vi "ConfigUI.vi"() -> ()   [LabVIEW 2017, in "ThreePhasePLL editor node.lvclass"]
uses:
  ThreePhasePLL editor node.lvclass
  <vilib>/NI/Configuration Framework/Node/NodeRef.ctl
  <vilib>/NI/Configuration Framework/Node/NISE_CEF_Node.lvclass
  <vilib>/NI/AMC/Message Queue.ctl
  <vilib>/NI/AMC/Message.ctl
  <vilib>/NI/Tools/Keyed Array/KeyedArray.ctl
  <vilib>/NI/Configuration Framework/Node/UserEventRef.ctl
  <vilib>/NI/Configuration Framework/Controls/EventCluster.ctl
  <vilib>/NI/Configuration Framework/Node/RefreshUIEvent.ctl
  <vilib>/NI/Configuration Framework/Node/CacheState.ctl
  <vilib>/NI/Configuration Framework/Node/StopEvent.ctl
  <vilib>/NI/Configuration Framework/Node/NodeChangeEvent.ctl
  <vilib>/NI/DCAF/Tag Editor Core/control module/configuration/error classification setting.ctl
  <vilib>/NI/Tag Bus Module Framework/runtime/error classification.ctl
  <vilib>/NI/DCAF/Tag Editor Core/Table API/Available Tag Menu/channel action event.ctl
  <vilib>/NI/DCAF/Tag Editor Core/Table API/Available Tag Menu/dialog output action.ctl
  <vilib>/NI/Tag Bus Module Framework/channel/TBM channel.lvclass
  <vilib>/NI/Tag Bus/tag/tag descriptor.lvclass
  <vilib>/NI/DCAF/Tag Editor Core/Table API/Table Manager/Call Back Ref Type Def.ctl
  <vilib>/NI/DCAF/Tag Editor Core/Configuration Editor/Classes/Engine Parent/Engine Parent Editor Node.lvclass
  <vilib>/NI/DCAF/Tag Editor Core/Configuration Editor/Classes/Module editor node/module editor node.lvclass
  C:/Program Files (x86)/National Instruments/LabVIEW 2017/vi.lib/NI/Configuration Framework/serializable node/NISE_CEF_serializable node.lvclass
  <vilib>/rvi/Analysis/control/PID/Typedef/niFpgaPID_PIGains.ctl
  <vilib>/rvi/Analysis/control/PID/Typedef/niFpgaPID_OutputRange.ctl
  <vilib>/NI/DCAF/Tag Editor Core/Table API/Table Manager/references.ctl
  <vilib>/NI/DCAF/Tag Editor Core/Table API/Table Manager/Menu Definition.ctl
  <vilib>/NI/DCAF/Tag Editor Core/Table API/Table Manager/Menu Options.ctl
  <vilib>/NI/DCAF/Tag Editor Core/control module/configuration/control module configuration.lvclass
  C:/Program Files (x86)/National Instruments/LabVIEW 2017/vi.lib/NI/Configuration Framework/serializable configuration/NISE_CEF_serializable configuration.lvclass
  <vilib>/NI/DCAF/Tag Editor Core/control module/editor node/control module editor.lvclass
  module/configuration/ThreePhasePLL configuration.lvclass
  C:/Program Files (x86)/National Instruments/LabVIEW 2017/vi.lib/NI/DCAF/Tag Editor Core/control module/configuration/control module configuration.lvclass
  module/configuration/ThreePhasePLL configuration.lvclass/ThreePhasePLL configuration.ctl
  <vilib>/NI/DCAF/Tag Editor Core/control module/configuration/control module configuration.lvclass/control module configuration.ctl
  <vilib>/NI/Configuration Framework/serializable configuration/NISE_CEF_serializable configuration.lvclass/NISE_CEF_serializable configuration.ctl
  <vilib>/NI/PowerElectronicsControl/ThreePhasePLL/Interface/Configuration.ctl
  <vilib>/NI/Tag Bus Module Framework/channel/channel classification.ctl
  <vilib>/NI/DCAF/Tag Editor Core/control module/configuration/Write error classifications.vi
  <vilib>/NI/Tag Bus Module Framework/module configuration/TBM module configuration.lvclass
  <vilib>/NI/DCAF/Tag Editor Core/Configuration Editor/Classes/Module editor node/Read Module Configuration.vi
  <vilib>/NI/DCAF/Tag Editor Core/control module/editor node/read fixed channel configuration.vi
  <vilib>/Utility/LVClass/Get LV Class Name.vi
  <vilib>/NI/Configuration Framework/error generator/NISE_error generator.vi
  <vilib>/NI/Configuration Framework/serializable configuration/NISE_CEF_serializable configuration.lvclass
  <vilib>/NI/DCAF/Tag Editor Core/Table API/Listbox/Multi Column Listbox.lvclass
  <vilib>/NI/Configuration Framework/NISE_CEF_TreeControl.lvlib
  <vilib>/NI/DCAF UI Toolkit/Controls/DCAF UI Elements.lvlib
  <vilib>/NI/Tools/Keyed Array/Tools_KeyedArray.lvlib
  <vilib>/NI/AMC/AMC.lvlib
  <vilib>/NI/DCAF/Tag Editor Core/Table API/Table Manager/Table Manager.lvclass
  <vilib>/NI/DCAF/Tag Editor Core/Table API/Table Manager.lvlib
  <vilib>/NI/PowerElectronicsControl/ThreePhasePLL/Interface/ThreePhasePLLInterface.lvlib
  <vilib>/NI/Tag Bus Module Framework/runtime/TBM module execution interface.lvclass
panel:
  in  "Enum":i32
  in  "Top Level Tab Control":T1(tab)
  in  "freqBoundaries":sgl caption="Frequency Boundaries (radians per second)"
  in  "lockDuration":sgl caption="Lock Duration (seconds)"
  in  "expectedFreq":sgl caption="Expected Frequency (radians per second)"
  in  "dT":sgl
  in  "PLL range":T2={"output high (Inf)"=inf, "output low (-Inf)"=-inf}
  in  "PLL gains":T3 {"proportional gain" step=0.125}
  in  "Channels Listbox":i32(listbox)
  in  "mapall":bool
  in  "mapwriters":bool
  in  "Parameters Listbox":i32(listbox)
  in  "error classifications":T4[](array[typedef])
  in  "user event out":refnum<user-event>
  in  "node change":T6
  in  "stop event":T7
  in  "cache state":T8
  in  "refresh UI":T9
  in  "user event":T10
  in  "main queue":T11
  in  "node ref":T12
  # "dT =  the rate of PLL execution in seconds\nExpected Frequency = Frequency expected to be locked onto (i.e. 50 Hz = 314.159 & 60 Hz = 376.991)\nLock Duration = the amount of time the detected frquency must be within Expected Frequency +/- Frequency Boundaries inorder to turn Locked to True\nFrequency Boundaries = the range Detected Frequency is allowed to diviate from the Expected Frequency and still be considered Locked"
  # "(Single-Click to Edit)"
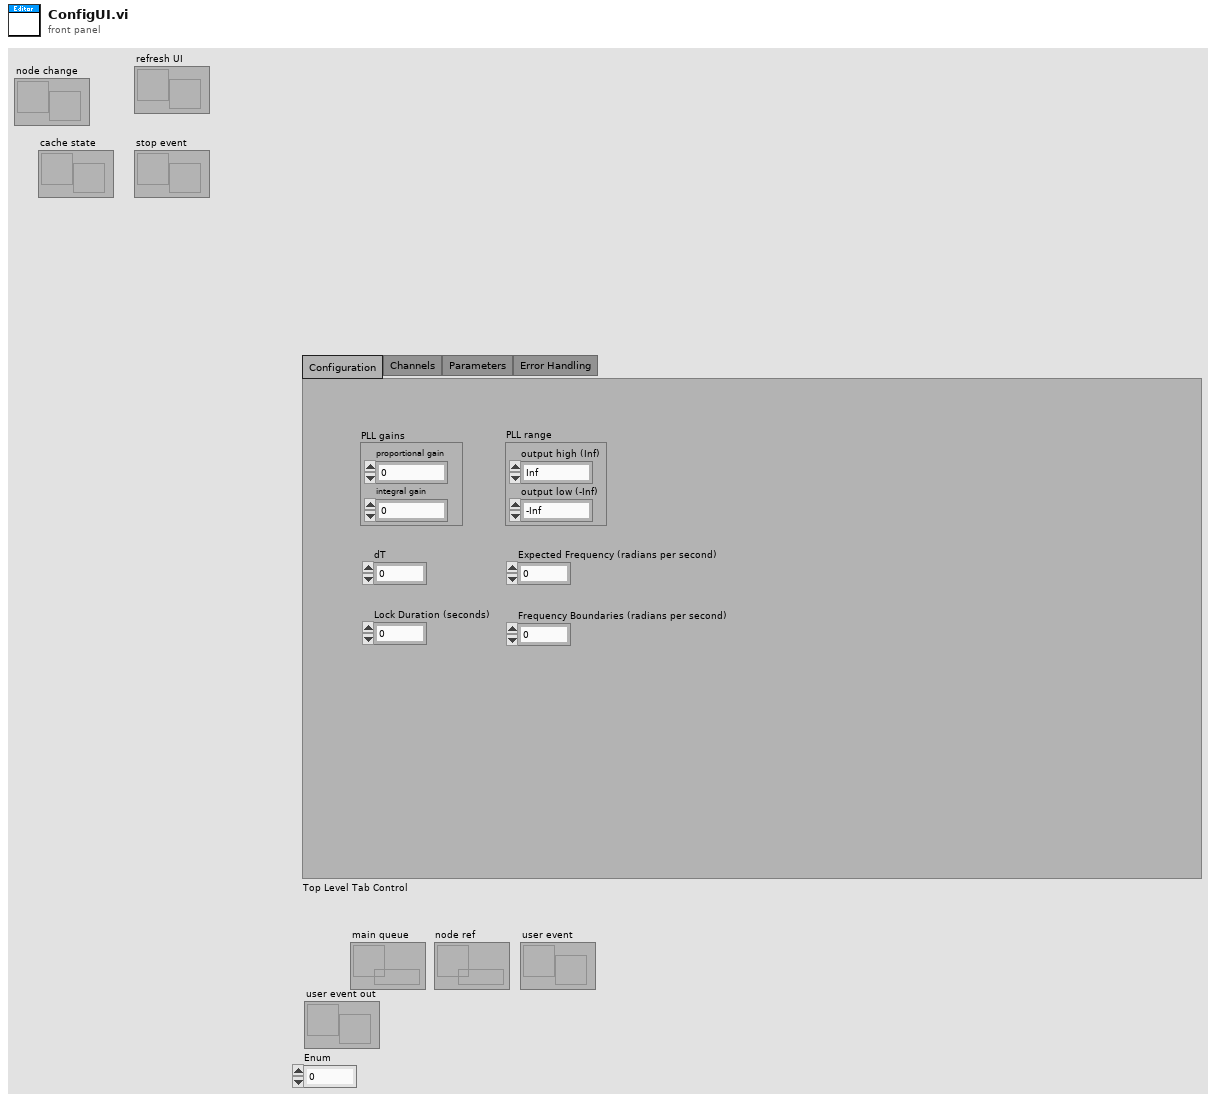
[diagram p1: front panel]
types:
  T1 = enum32{"Configuration", "Channels", "Parameters", "Error Handling"}
  T2 = typedef "niFpgaPID_OutputRange.ctl" = cluster{"output high (Inf)":sgl, "output low (-Inf)":sgl}
  T3 = typedef "niFpgaPID_PIGains.ctl" = cluster{"proportional gain":sgl, "integral gain":sgl}
  T4 = typedef "control module configuration.lvclass/error classification setting.ctl" = cluster{"code":i32, "error classification":T5}
  T5 = typedef "TBM module execution interface.lvclass/error classification.ctl" = enum16{"unknown", "none", "trivial", "recoverable", "critical"}
  T6 = typedef "NISE_CEF_Node.lvclass/NodeChangeEvent.ctl" = refnum<user-event>
  T7 = typedef "NISE_CEF_Node.lvclass/StopEvent.ctl" = refnum<user-event>
  T8 = typedef "NISE_CEF_Node.lvclass/CacheState.ctl" = refnum<user-event>
  T9 = typedef "NISE_CEF_Node.lvclass/RefreshUIEvent.ctl" = refnum<user-event>
  T10 = typedef "NISE_CEF_Node.lvclass/UserEventRef.ctl" = refnum<user-event>
  T11 = typedef "AMC.lvlib/Message Queue.ctl" = refnum<queue>
  T12 = typedef "NISE_CEF_Node.lvclass/NodeRef.ctl" = refnum<data-value>
  T13 = typedef "Table Manager.lvlib/Table Manager.lvclass/Menu Definition.ctl" = cluster{"Menu Name":string, "Menu Options":T14}
  T14 = typedef "Table Manager.lvlib/Table Manager.lvclass/Menu Options.ctl" = enum16{"Always Show", "Show When Used", "Show When Empty"}
  T15 = typedef "Table Manager.lvlib/Table Manager.lvclass/references.ctl" = cluster{"stop event":T7, "refresh UI":T9, "cache state":T8, "node change":T6, "user event out":refnum<user-event>, "main queue":T11, "user event":T10}
  T16 = typedef "Table Manager.lvlib/Column.lvclass/Column Descriptor.ctl" = cluster{"name":string, "caption":string, "Column Type":T17, "Params":string, "AutoSizeMode":i32, "FillWeight":sgl, "MinWidth":u32, "tooltip":string, "Enum Reference":refnum<vi>, "Channel suffix":string, "Read Only":bool, "Call Back VI":T18, "DT Dependency":i32, "name dependency":i32, "data type":T19, "Custom Column":refnum<class "Column.lvclass">}
  T17 = typedef "Table Manager.lvlib/Column.lvclass/Column Type.ctl" = enum16{"String", "Mapping", "Enum", "Custom"}
  T18 = typedef "Table Manager.lvlib/Table Manager.lvclass/Call Back Ref Type Def.ctl" = refnum<vi>
  T19 = typedef "tag bus.lvlib/tag descriptor.lvclass/Data Type.ctl" = enum16{"Double", "Single", "I64", "I32", "I16", "I8", "U64", "U32", "U16", "U8", "Boolean", "String", "Array of Double", "Array of Single", "Array of I64", "Array of I32", "Array of I16", "Array of I8", "Array of U64", "Array of U32", "Array of U16", "Array of U8", "Array of Boolean", "Array of String"}
  T20 = typedef "Table Manager.lvlib/Table Manager.lvclass/object ref.ctl" = cluster{"engine":refnum<data-value>, "Node Ref":refnum<data-value>}
  T21 = typedef "Table Manager.lvlib/Table Manager.lvclass/Table Events.ctl" = cluster{"Menu Selection":refnum<user-event>}
  T22 = typedef "NISE_CEF_TreeControl.lvlib/EventCluster.ctl" = cluster{"command":string, "data":string}
  T23 = typedef "ThreePhasePLLInterface.lvlib/Configuration.ctl" = cluster{"PLLgains":T3, "PLLrange":T2, "dT":sgl, "expectedFreq":sgl, "lockDuration":sgl, "freqBoundaries":sgl}
  T24 = typedef "TBM channel.lvclass/channel classification.ctl" = enum16{"input data", "output data", "processing parameter", "processing result"}
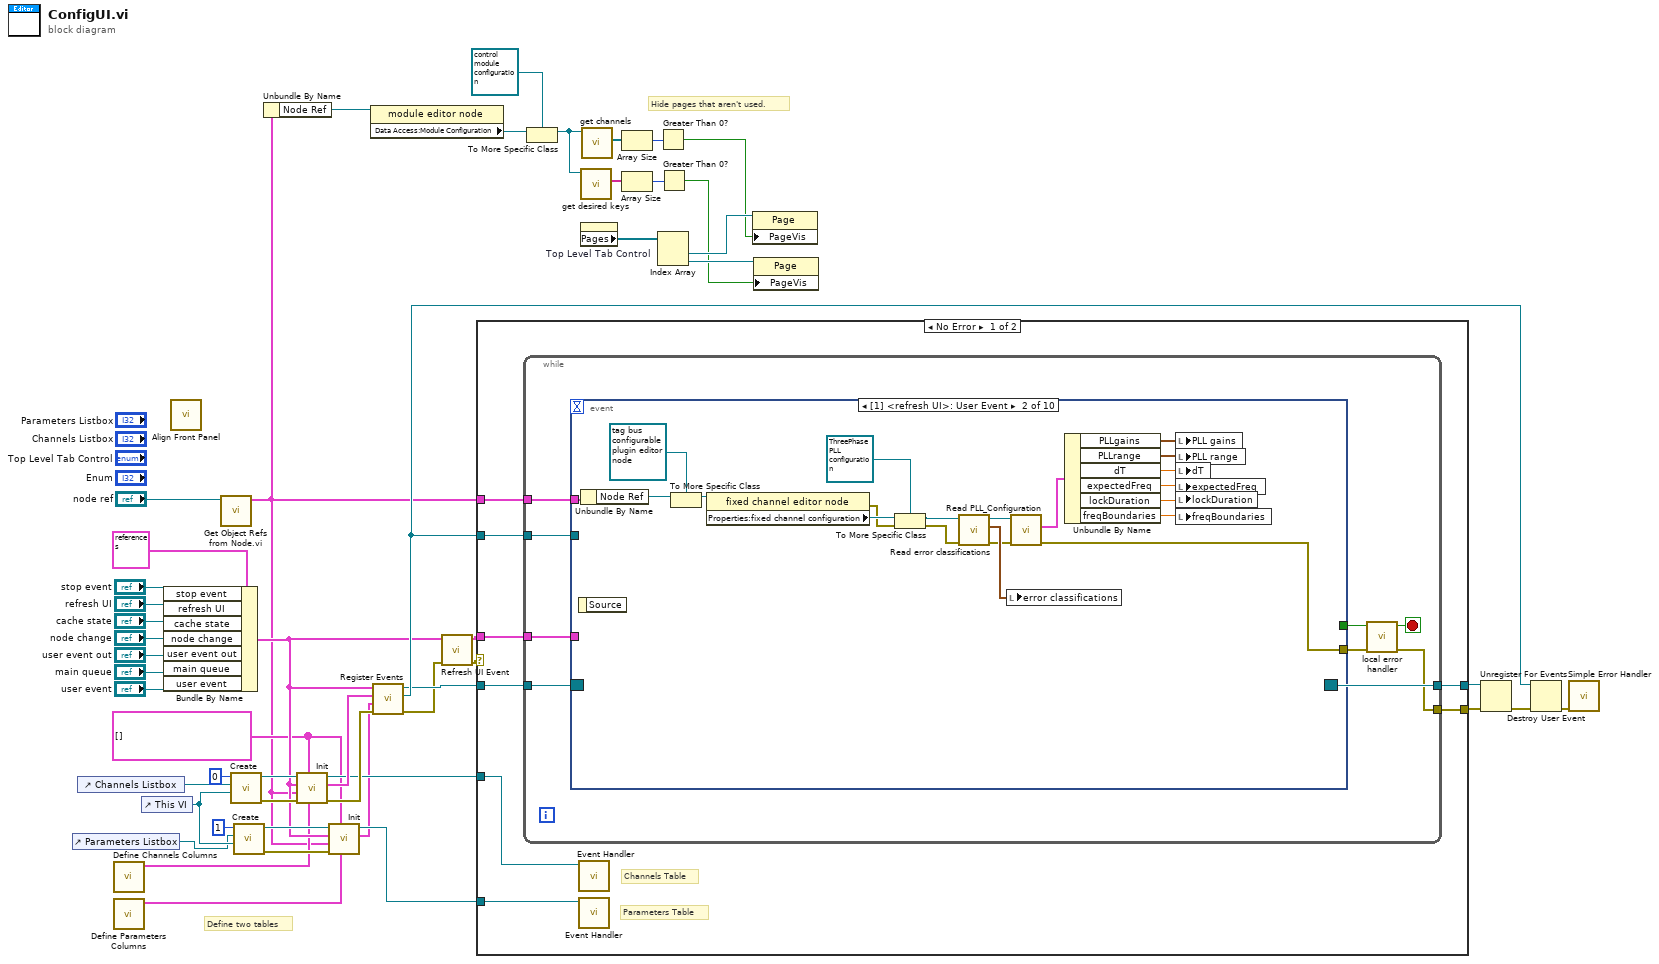
[diagram p0: block diagram]
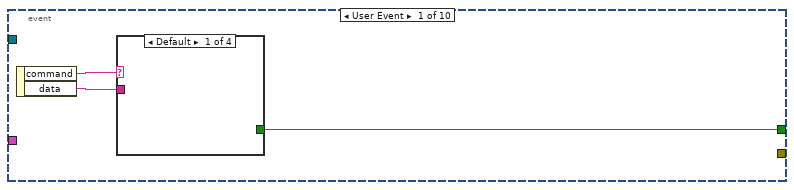
[diagram p2: hidden frame]
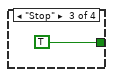
[diagram p4: hidden frame]
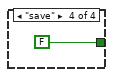
[diagram p5: hidden frame]
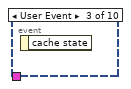
[diagram p6: hidden frame]
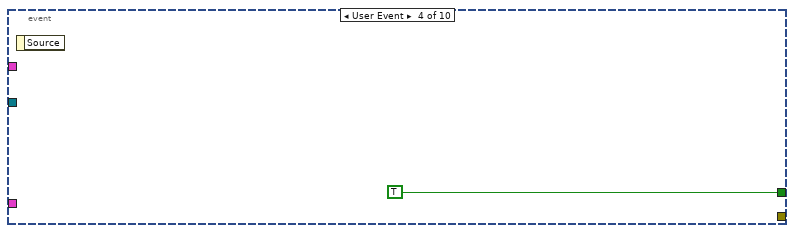
[diagram p7: hidden frame]
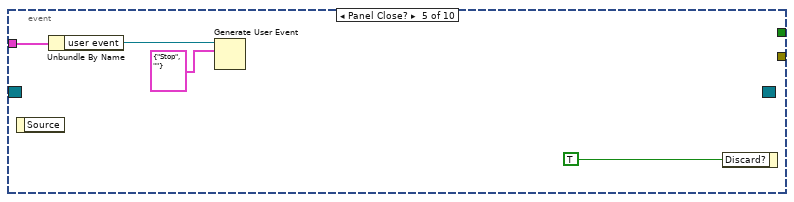
[diagram p8: hidden frame]
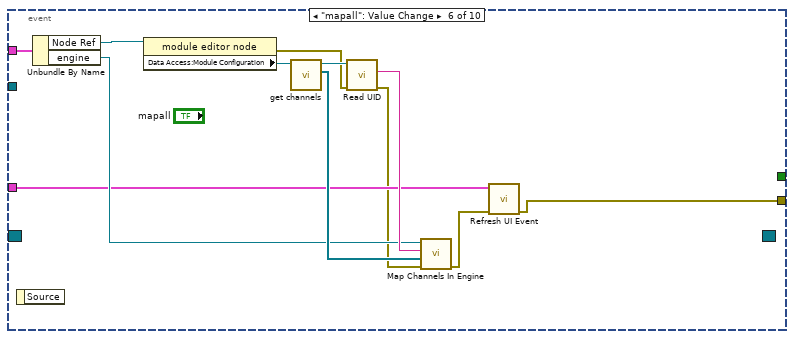
[diagram p9: hidden frame]
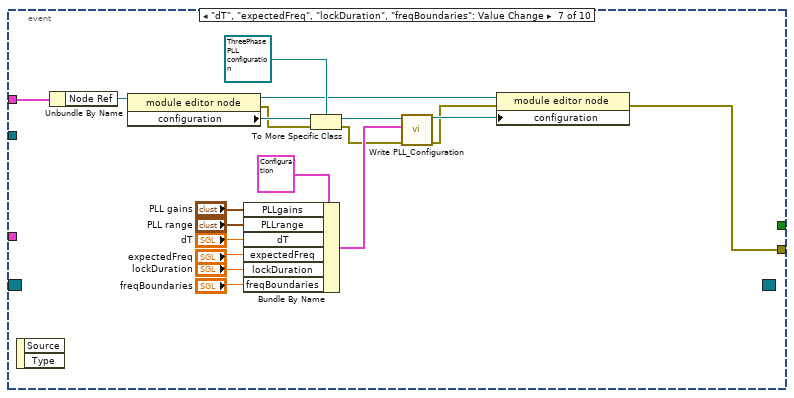
[diagram p10: hidden frame]
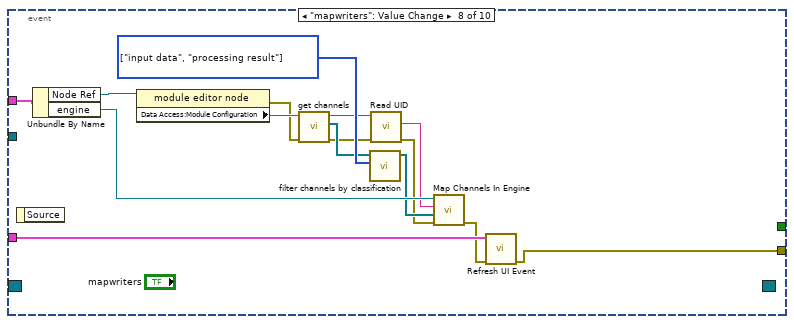
[diagram p11: hidden frame]
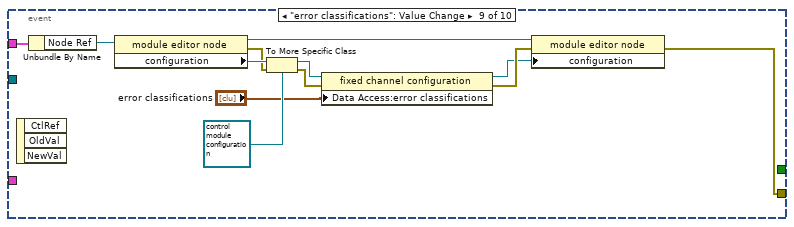
[diagram p12: hidden frame]
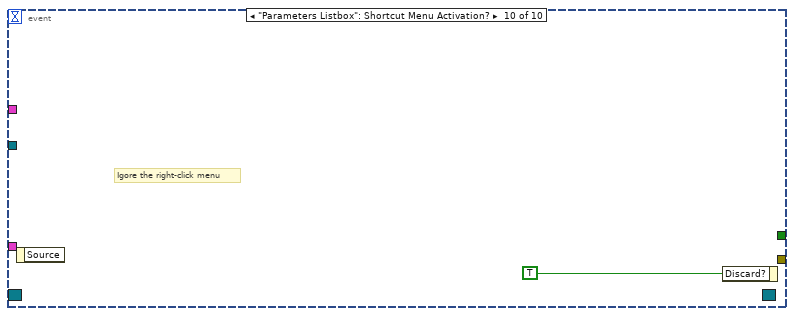
[diagram p13: hidden frame]
diagram:
  w15 = T13[] [] ("Right-Click Menu")
  # "Define two tables"
  # "Hide pages that aren't used."
  n1 = control-ref of="Parameters Listbox"() -> (w18:refnum<vi>)
  n2 = control-ref of="Channels Listbox"() -> (w26:refnum<vi>)
  n3 = call <vilib>:"Define Channels Columns.vi"() -> ("Column Descriptors"=w17:T16[])  [unwired: 11 in]
  n4 = call <vilib>:"Define Parameters Columns.vi"() -> ("Column Descriptors"=w16:T16[])  [unwired: 11 in]
  n5 = control-ref of="This VI"() -> (w22:refnum<vi>)
  n6 = Bundle By Name(cluster=T15 {"stop event"=refnum, "refresh UI"=refnum, "cache state"=refnum, "node change"=refnum, "user event out"=refnum, "main queue"=refnum, "user event"=refnum} ("Event References"), "stop event"="stop event", "refresh UI"="refresh UI", "cache state"="cache state", "node change"="node change", "user event out"="user event out", "main queue"="main queue", "user event"="user event") -> (w19:T15)
  n7 = call <vilib>:"Align Front Panel.vi"() -> ()  [unwired: 10 in, 2 out]
  n8 = call <vilib>:"Get Object Refs from Node.vi.vi"("node ref"="node ref") -> ("Node object refs"=w7:T20)  [unwired: 9 in, 1 out]
  n9 = call <vilib>:"Create.vi"("Top VI"=w22, "Listbox"=w26, "Index"=0) -> ("error out"=w29:errorcluster, "reference out"=w30:refnum<class "Multi Column Listbox.lvclass">)  [unwired: 7 in]
  n10 = call <vilib>:"Create.vi"("Top VI"=w22, "Listbox"=w18, "Index"=1) -> ("error out"=w25:errorcluster, "reference out"=w24:refnum<class "Multi Column Listbox.lvclass">)  [unwired: 7 in]
  n11 = Unbundle By Name(w7) -> ("Node Ref"=w5:refnum<data-value>)
  n12 = call-dynamic "Init.vi"("Column Descriptors"=w17, "Right-Click Menu"=w15, "error in (no error)"=w29, "Node object refs"=w7, "Event References"=w19, "Multi Column Listbox in"=w30) -> ("error out"=w28:errorcluster, "Table Events"=w40:T21, "Multi Column Listbox out"=w27:refnum<class "Multi Column Listbox.lvclass">)  [unwired: 3 in]
  n13 = call-dynamic "Init.vi"("Column Descriptors"=w16, "Right-Click Menu"=w15, "error in (no error)"=w25, "Node object refs"=w7, "Event References"=w19, "Multi Column Listbox in"=w24) -> ("Table Events"=w20:T21, "Multi Column Listbox out"=w21:refnum<class "Multi Column Listbox.lvclass">)  [unwired: 3 in, 1 out]
  n14 = property class="module editor node"(reference=w5) -> ("Data Access:Module Configuration"=w6:refnum<class "TBM module configuration.lvclass">)  [unwired: 1 in, 2 out]
  n15 = call <vilib>:"Register Events.vi"("error in (no error)"=w28, "Parameters Table Events"=w20, "Channels Table Events"=w40, "Event References"=w19) -> ("error out"=w33:errorcluster, "Channel Action"=w39:refnum<user-event>, "Event Registration Refnum"=w38:refnum<event-registration>)  [unwired: 5 in]
  n16 = call <vilib>:"Refresh UI Event.vi"("error in (no error)"=w33, "Event References"=w19) -> ("error out"=w34:errorcluster, "Event References out"=w32:T15)  [unwired: 8 in]
  n17 = case shown="No Error" w34 {
    selector: w34 -> [_ w157]
    tunnel: w38 -> [w58 w156]
    tunnel: [w57 w156] -> w50
    tunnel: [w55 w157] -> w49
    tunnel: w39 -> [w56 _]
    tunnel: w7 -> [w54 _]
    tunnel: w32 -> [w53 _]
    tunnel: w27 -> [w52 _]
    tunnel: w21 -> [w51 _]
    frame No Error {
      # "Parameters Table"
      # "Channels Table"
      n18 = while {
        tunnel: w58 -> [w67]
        tunnel: [w66] -> w57
        tunnel: w56 -> [w65]
        tunnel: [w61] -> w55
        tunnel: w54 -> [w60]
        tunnel: w53 -> [w59]
        stop <- w63 stop-if-true
        n19 = event shown="[1] <refresh UI>: User Event" {
          selector: w67 -> [_ _ _ _ _ _ _ _ _ _]
          dyn-events: [_ _ _ _ _ _ _ _ _ _] -> w66
          timeout: _ -> [_ _ _ _ _ _ _ _ _ _]
          tunnel: [w70 _ _ TRUE _ _ _ _ _ _] -> w64
          tunnel: [_ w79 _ _ _ w103 w110 w138 w154 _] -> w62
          tunnel: w65 -> [_ _ _ _ _ _ _ _ _ _]
          tunnel: w60 -> [_ w92 _ _ _ w107 w121 w139 w153 _]
          tunnel: w59 -> [_ _ _ _ w95 w102 _ w137 _ _]
          event User Event {
            n20 = event-data() -> ("command"=w69:string, "data"=w68:string)  [unwired: 1 in]
            n21 = case shown="Default" w69 {
              tunnel: [_ _ TRUE FALSE] -> w70
              tunnel: w68 -> [_ _ _ _]
              frame Default {
              }
              frame "Refresh" {
              }
              frame "Stop" {
              }
              frame "save" {
              }
            }
          }
          event User Event {
            n22 = event-data() -> ()  [unwired: 1 in, 1 out]
            n23 = Unbundle By Name(w92) -> ("Node Ref"=w90:refnum<data-value>)
            n24 = To More Specific Class(target class=refnum<data-value> refnum ("data value reference"), reference=w90) -> (specific class reference=w89:refnum<data-value>)  [unwired: 1 in, 1 out]
            n25 = property class="fixed channel editor node"(reference=w89) -> (error out=w85:errorcluster, "Properties:fixed channel configuration"=w87:refnum<class "control module configuration.lvclass">)  [unwired: 1 in, 1 out]
            n26 = To More Specific Class(target class=refnum<class "ThreePhasePLL configuration.lvclass"> refnum ("ThreePhasePLL configuration"), reference=w87, error in=w85) -> (specific class reference=w86:refnum<class "ThreePhasePLL configuration.lvclass">, error out=w84:errorcluster)
            n27 = call <vilib>:"Read error classifications.vi"("error in"=w84, "control module configuration in"=w86) -> ("error out"=w81:errorcluster, "error classifications"=w88:T4[], "control module configuration out"=w82:refnum<class "ThreePhasePLL configuration.lvclass">)  [unwired: 7 in]
            n28 = local write "error classifications"(w88) -> ()
            n29 = call "Read PLL_Configuration.vi"("error in (no error)"=w81, "ThreePhasePLL configuration in"=w82) -> ("error out"=w79:errorcluster, "Configuration"=w80:T23)  [unwired: 7 in, 1 out]
            n30 = Unbundle By Name(w80) -> ("PLLgains"=w78:T3, "PLLrange"=w77:T2, "dT"=w76:sgl, "expectedFreq"=w75:sgl, "lockDuration"=w74:sgl, "freqBoundaries"=w73:sgl)
            n31 = local write "PLL gains"(w78) -> ()
            n32 = local write "PLL range"(w77) -> ()
            n33 = local write "dT"(w76) -> ()
            n34 = local write "expectedFreq"(w75) -> ()
            n35 = local write "lockDuration"(w74) -> ()
            n36 = local write "freqBoundaries"(w73) -> ()
          }
          event User Event {
            n37 = event-data() -> ()  [unwired: 1 in, 1 out]
          }
          event User Event {
            n38 = event-data() -> ()  [unwired: 1 in, 1 out]
          }
          event Panel Close? {
            n39 = event-data() -> ()  [unwired: 1 in, 1 out]
            n40 = Unbundle By Name(w95) -> ("user event"=w94:T10)
            n41 = Generate User Event(user event=w94, event data cluster=T22 {"command"="Stop", "data"=""} ("event data")) -> ()  [unwired: 2 in, 2 out]
            n42 = event-data("Discard?"=TRUE) -> ()  [unwired: 1 in, 1 out]
          }
          event "mapall": Value Change {
            n43 = event-data() -> ()  [unwired: 1 in, 1 out]
            n44 = Unbundle By Name(w107) -> ("Node Ref"=w106:refnum<data-value>, "engine"=w105:refnum<data-value>)
            n45 = property class="module editor node"(reference=w106) -> (error out=w99:errorcluster, "Data Access:Module Configuration"=w101:refnum<class "TBM module configuration.lvclass">)  [unwired: 1 in, 1 out]
            n46 = call-dynamic "get channels.vi"("module configuration in"=w101) -> ("channels"=w109:refnum<class "TBM channel.lvclass">[], "module configuration out"=w100:refnum<class "TBM module configuration.lvclass">)  [unwired: 9 in]
            n47 = call <vilib>:"Read UID.vi"("error in"=w99, "configuration in"=w100) -> ("error out"=w98:errorcluster, "instance id"=w108:string)  [unwired: 7 in, 1 out]
            n48 = call <vilib>:"Map Channels In Engine.vi"("error in (no error)"=w98, "channels"=w109, "instance id"=w108, "Engine DVR"=w105) -> ("error out"=w104:errorcluster)  [unwired: 7 in]
            n49 = call <vilib>:"Refresh UI Event.vi"("error in (no error)"=w104, "Event References"=w102) -> ("error out"=w103:errorcluster)  [unwired: 8 in, 1 out]
          }
          event "dT", "expectedFreq", "lockDuration", "freqBoundaries": Value Change {
            n50 = event-data() -> ()  [unwired: 1 in, 2 out]
            n51 = Unbundle By Name(w121) -> ("Node Ref"=w120:refnum<data-value>)
            n52 = property class="module editor node"(reference=w120) -> (reference out=w115:refnum<data-value>, error out=w113:errorcluster, "configuration"=w119:refnum<class "NISE_CEF_serializable configuration.lvclass">)  [unwired: 1 in]
            n53 = Bundle By Name(cluster=T23 {"PLLgains"={"proportional gain"=0.0, "integral gain"=0.0}, "PLLrange"={"output high (Inf)"=inf, "output low (-Inf)"=-inf}, "dT"=0.0, "expectedFreq"=0.0, "lockDuration"=0.0, "freqBoundaries"=0.0} ("Configuration"), "PLLgains"="PLL gains", "PLLrange"="PLL range", "dT"="dT", "expectedFreq"="expectedFreq", "lockDuration"="lockDuration", "freqBoundaries"="freqBoundaries") -> (w116:T23)
            n54 = To More Specific Class(target class=refnum<class "ThreePhasePLL configuration.lvclass"> refnum ("ThreePhasePLL configuration"), reference=w119, error in=w113) -> (specific class reference=w117:refnum<class "ThreePhasePLL configuration.lvclass">, error out=w112:errorcluster)
            n55 = call "Write PLL_Configuration.vi"("error in (no error)"=w112, "Configuration"=w116, "ThreePhasePLL configuration in"=w117) -> ("error out"=w111:errorcluster, "ThreePhasePLL configuration out"=w114:refnum<class "ThreePhasePLL configuration.lvclass">)  [unwired: 7 in]
            n56 = property class="module editor node"(reference=w115, error in=w111, "configuration"=w114) -> (error out=w110:errorcluster)  [unwired: 1 out]
          }
          event "mapwriters": Value Change {
            w142 = T24[] [enum."input data", enum."processing result"] items=["input data", "output data", "processing parameter", "processing result"] ("allowed classifications")
            n57 = event-data() -> ()  [unwired: 1 in, 1 out]
            n58 = Unbundle By Name(w139) -> ("Node Ref"=w140:refnum<data-value>, "engine"=w136:refnum<data-value>)
            n59 = property class="module editor node"(reference=w140) -> (error out=w129:errorcluster, "Data Access:Module Configuration"=w131:refnum<class "TBM module configuration.lvclass">)  [unwired: 1 in, 1 out]
            n60 = call-dynamic "get channels.vi"("module configuration in"=w131) -> ("channels"=w141:refnum<class "TBM channel.lvclass">[], "module configuration out"=w130:refnum<class "TBM module configuration.lvclass">)  [unwired: 9 in]
            n61 = call <vilib>:"filter channels by classification.vi"("allowed classifications"=w142, "channels in"=w141) -> ("channels out"=w134:refnum<class "TBM channel.lvclass">[])  [unwired: 9 in]
            n62 = call <vilib>:"Read UID.vi"("error in"=w129, "configuration in"=w130) -> ("error out"=w133:errorcluster, "instance id"=w135:string)  [unwired: 7 in, 1 out]
            n63 = call <vilib>:"Map Channels In Engine.vi"("error in (no error)"=w133, "channels"=w134, "instance id"=w135, "Engine DVR"=w136) -> ("error out"=w132:errorcluster)  [unwired: 7 in]
            n64 = call <vilib>:"Refresh UI Event.vi"("error in (no error)"=w132, "Event References"=w137) -> ("error out"=w138:errorcluster)  [unwired: 8 in, 1 out]
          }
          event "error classifications": Value Change {
            n65 = event-data() -> ()  [unwired: 1 in, 3 out]
            n66 = Unbundle By Name(w153) -> ("Node Ref"=w148:refnum<data-value>)
            n67 = property class="module editor node"(reference=w148) -> (reference out=w152:refnum<data-value>, error out=w144:errorcluster, "configuration"=w147:refnum<class "NISE_CEF_serializable configuration.lvclass">)  [unwired: 1 in]
            n68 = To More Specific Class(target class=refnum<class "control module configuration.lvclass"> refnum ("fixed channel configuration"), reference=w147, error in=w144) -> (specific class reference=w149:refnum<class "control module configuration.lvclass">, error out=w143:errorcluster)
            n69 = property class="fixed channel configuration"(reference=w149, error in=w143, "Data Access:error classifications"="error classifications") -> (reference out=w150:refnum<class "control module configuration.lvclass">, error out=w151:errorcluster)
            n70 = property class="module editor node"(reference=w152, error in=w151, "configuration"=w150) -> (error out=w154:errorcluster)  [unwired: 1 out]
          }
          event "Parameters Listbox": Shortcut Menu Activation? {
            # "Igore the right-click menu"
            n71 = event-data() -> ()  [unwired: 1 in, 1 out]
            n72 = event-data("Discard?"=TRUE) -> ()  [unwired: 1 in, 1 out]
          }
        }
        n73 = call <vilib>:"local error handler.vi"("error in (no error)"=w62, "Stop in"=w64) -> ("error out"=w61:errorcluster, "Stop out"=w63:bool)  [unwired: 8 in]
      }
      n74 = call-dynamic "Event Handler.vi"("Listbox in"=w52) -> ()  [unwired: 9 in, 2 out]
      n75 = call-dynamic "Event Handler.vi"("Listbox in"=w51) -> ()  [unwired: 9 in, 2 out]
    }
    frame Error {
    }
  }
  n76 = To More Specific Class(target class=refnum<class "control module configuration.lvclass"> refnum ("fixed channel configuration"), reference=w6) -> (specific class reference=w3:refnum<class "control module configuration.lvclass">)  [unwired: 1 in, 1 out]
  n77 = call-dynamic "get desired keys.vi"("fixed channel configuration in"=w3) -> ("desired keys"=w11:string[])  [unwired: 8 in, 2 out]
  n78 = property on="Top Level Tab Control" class="TabCtl (strict)"() -> ("Pages"=w8:refnum<vi>[])  [unwired: 2 in, 2 out]
  n79 = call-dynamic "get channels.vi"("fixed channel configuration in"=w3) -> ("channels"=w14:refnum<class "TBM channel.lvclass">[])  [unwired: 9 in, 1 out]
  n80 = Array Size(array=w14) -> (size(s)=w13:i32)
  n81 = Array Size(array=w11) -> (size(s)=w12:i32)
  n82 = Greater Than 0?(x=w13) -> (x > 0?=w2:bool)
  n83 = Index Array(array=w8) -> (element #1=w9:refnum<vi>, element #2=w10:refnum<vi>)  [unwired: 2 in]
  n84 = Greater Than 0?(x=w12) -> (x > 0?=w1:bool)
  n85 = property class="Page"(reference=w9, "PageVis"=w2) -> ()  [unwired: 1 in, 2 out]
  n86 = property class="Page"(reference=w10, "PageVis"=w1) -> ()  [unwired: 1 in, 2 out]
  n87 = Unregister For Events(event registration refnum=w50, error in=w49) -> (error out=w48:errorcluster)
  n88 = Destroy User Event(user event=w39, error in=w48) -> (error out=w47:errorcluster)
  n89 = call <vilib>:"Simple Error Handler.vi"("error in (no error)"=w47) -> ()  [unwired: 4 in, 5 out]
